vi "Previous Element Sum.vi"() -> ()   [LabVIEW 2025]
panel:
  out "Output Array":dbl[](array[numeric])
  in  "Input Array":dbl[](array[numeric])
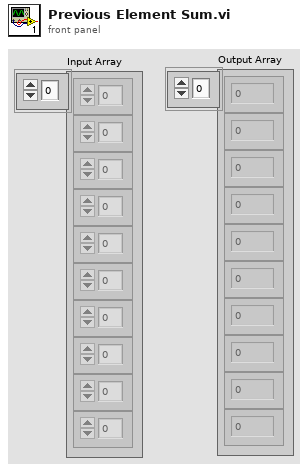
[diagram p1: front panel]
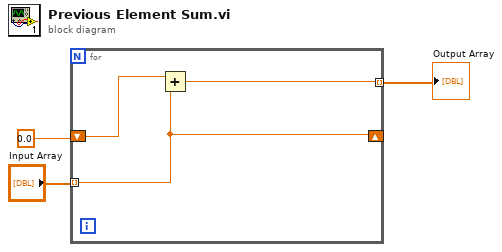
[diagram p0: block diagram]
diagram:
  n1 = for {
    tunnel: "Input Array" -> [w4] mode=indexing
    tunnel: [w6] -> w3 mode=indexing
    shift-right: [w4] -> _
    shift-left: 0.0 -> [w5]
    n2 = Add(x=w5, y=w4) -> (x+y=w6:dbl)
  }
  "Output Array" <- w3
